vi "3-2-4 gen random multi-data.vi"() -> (3 "output cluster":T1)   [LabVIEW 2020]
uses:
  <vilib>/numeric/Random Number (Range) DBL.vi
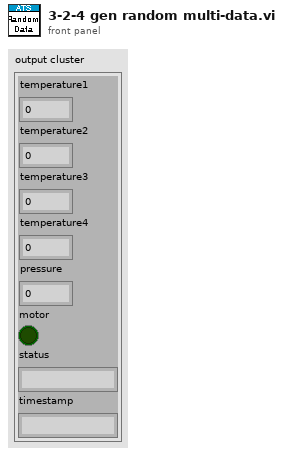
[diagram p1: front panel]
types:
  T1 = cluster{"temperature1":dbl, "temperature2":dbl, "temperature3":dbl, "temperature4":dbl, "pressure":dbl, "motor":bool, "status":string, "timestamp":string}
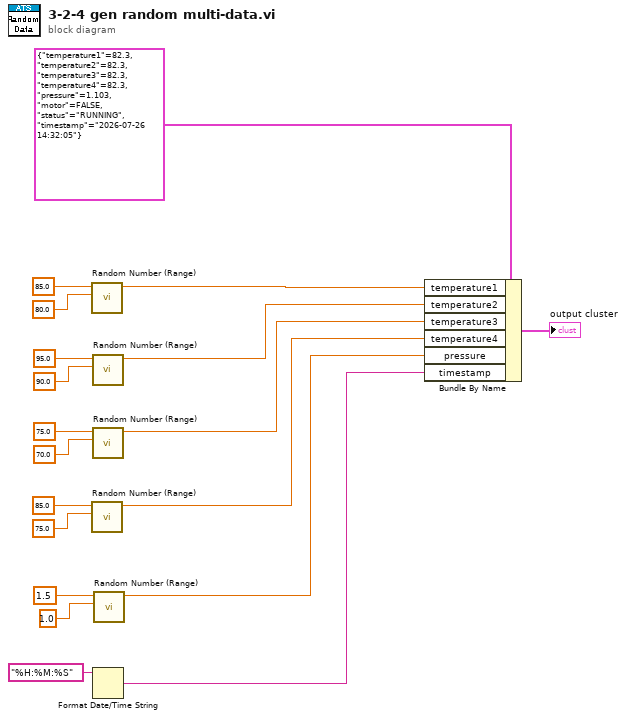
[diagram p0: block diagram]
diagram:
  n1 = call-poly <vilib>:"Random Number (Range).vi"("lower bound (0)"=80.0 ("upper bound (100)"), "upper bound (100)"=85.0) -> ("number"=w5:dbl)  [unwired: 9 in]
  n2 = call-poly <vilib>:"Random Number (Range).vi"("lower bound (0)"=75.0 ("upper bound (100)"), "upper bound (100)"=85.0) -> ("number"=w2:dbl)  [unwired: 9 in]
  n3 = call-poly <vilib>:"Random Number (Range).vi"("lower bound (0)"=90.0 ("upper bound (100)"), "upper bound (100)"=95.0) -> ("number"=w4:dbl)  [unwired: 9 in]
  n4 = call-poly <vilib>:"Random Number (Range).vi"("lower bound (0)"=70.0 ("upper bound (100)"), "upper bound (100)"=75.0) -> ("number"=w3:dbl)  [unwired: 9 in]
  n5 = Format Date/Time String(time format string (%c)="%H:%M:%S") -> (date/time string=w12:string)  [unwired: 2 in]
  n6 = call-poly <vilib>:"Random Number (Range).vi"("lower bound (0)"=1.0 ("upper bound (100)"), "upper bound (100)"=1.5) -> ("number"=w13:dbl)  [unwired: 9 in]
  n7 = Bundle By Name(cluster=T1 {"temperature1"=82.3, "temperature2"=82.3, "temperature3"=82.3, "temperature4"=82.3, "pressure"=1.103, "motor"=FALSE, "status"="RUNNING", "timestamp"="2026-07-26 14:32:05"} ("sensor_data"), "temperature1"=w5, "temperature2"=w4, "temperature3"=w3, "temperature4"=w2, "pressure"=w13, "timestamp"=w12) -> (→"output cluster":T1)
